vi "rotation_XY.vi"(3 "y_pos":dbl, 4 "x_pos":dbl, 5 "angle":dbl) -> (0 "rot_y":dbl, 1 "rot_x":dbl)   [LabVIEW 2012]
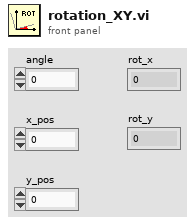
[diagram p1: front panel]
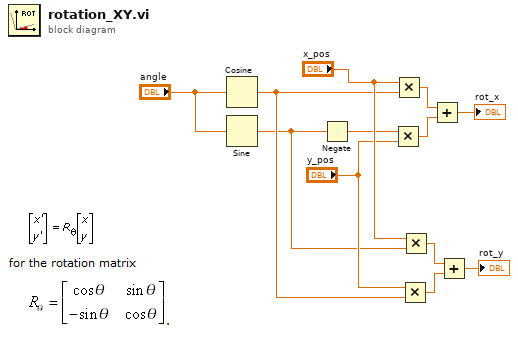
[diagram p0: block diagram]
diagram:
  n1 = Cosine(x="angle") -> (cos(x)=w3:dbl)
  n2 = Sine(x="angle") -> (sin(x)=w2:dbl)
  n3 = Negate(x=w2) -> (-x=w1:dbl)
  n4 = Multiply(x=w1, y="y_pos") -> (x*y=w11:dbl)
  n5 = Multiply(x="x_pos", y=w3) -> (x*y=w10:dbl)
  n6 = Multiply(x="y_pos", y=w3) -> (x*y=w6:dbl)
  n7 = Multiply(x="x_pos", y=w2) -> (x*y=w7:dbl)
  n8 = Add(x=w10, y=w11) -> (x+y=→"rot_x":dbl)
  n9 = Add(x=w7, y=w6) -> (x+y=→"rot_y":dbl)
